vi "SUB-Filter kalman.vi"(3 "x set":dbl[](array[numeric]) step=1.0) -> (1 "Kalman X":dbl[](array[numeric]) format="%.5f")   [LabVIEW 2015]
panel:
  out "P":dbl[](array[numeric])
  out "x":dbl[](array[numeric])
  # "칼만 필터"
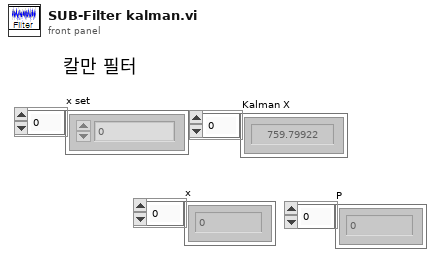
[diagram p1: front panel]
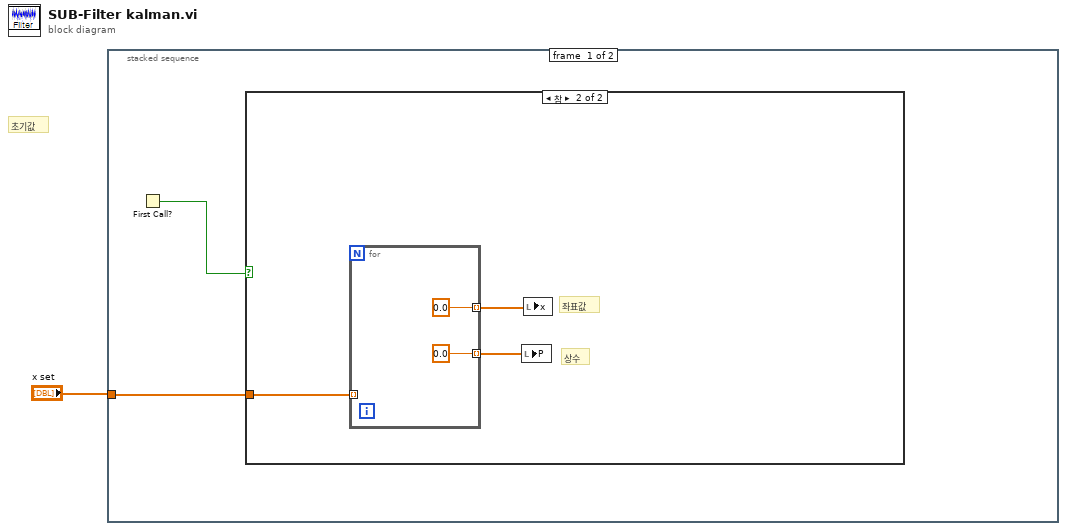
[diagram p0: block diagram]
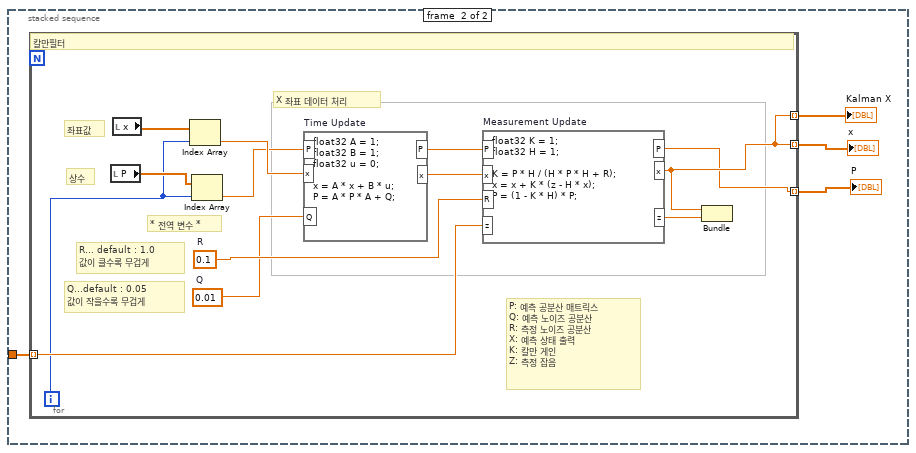
[diagram p3: hidden frame]
diagram:
  # "초기값"
  n1 = stacked-sequence {
    tunnel: "x set" -> [w2 w12]
    frame #0 {
      n2 = First Call?() -> (First Call?: T/F=w3:bool)
      n3 = case shown="참" w3 {
        tunnel: w2 -> [_ w6]
        frame False {
        }
        frame True {
          # "좌표값"
          # "상수"
          n4 = for {
            tunnel: w6 -> [_] mode=indexing
            tunnel: [0.0] -> w5 mode=indexing
            tunnel: [0.0] -> w4 mode=indexing
          }
          n5 = local write "P"(w4) -> ()
          n6 = local write "x"(w5) -> ()
        }
      }
    }
    frame #1 {
      n7 = for {
        tunnel: w12 -> [w20] mode=indexing
        tunnel: [w19] -> w11 mode=indexing
        tunnel: [w19] -> w10 mode=indexing
        tunnel: [w18] -> w9 mode=indexing
        i -> [w13]
        w24 = 0.01  # Q
        w25 = 0.1  # R
        # "좌표값"
        # "상수"
        # "P: 예측 공분산 매트릭스\nQ: 예측 노이즈 공분산\nR: 측정 노이즈 공분산\nX: 예측 상태 출력 \nK: 칼만 게인\nZ: 측정 잡음"
        # "X 좌표 데이터 처리"
        # "* 전역 변수 *"
        # "Q...default : 0.05\n값이 작을수록 무겁게"
        # "R... default : 1.0\n값이 클수록 무겁게"
        # "칼만필터"
        n8 = local read "P"() -> (w14:dbl[])
        n9 = local read "x"() -> (w17:dbl[])
        n10 = Index Array(array=w17, index=w13) -> (element=w16:dbl)
        n11 = Index Array(array=w14, index=w13) -> (element=w15:dbl)
        n12 = formula code="float32 A = 1;\nfloat32 B = 1;\nfloat32 u = 0;\n\nx = A * x + B * u;\nP = A * P * A + Q;" "Time Update"("x"=w16, "P"=w15, "Q"=w24) -> ("x"=w23:dbl, "P"=w22:dbl)
        n13 = formula code="float32 K = 1;\nfloat32 H = 1;\n\nK = P * H / (H * P * H + R);\nx = x + K * (z - H * x);\nP = (1 - K * H) * P;" "Measurement Update"("x"=w23, "P"=w22, "z"=w20, "R"=w25) -> ("x"=w19:dbl, "P"=w18:dbl, "z"=w21:dbl)
        n14 = Bundle("x"=w19, "z"=w21) -> ()  [unwired: 1 in, 1 out]
      }
      "Kalman X" <- w11
      "x" <- w10
      "P" <- w9
    }
  }
